vi "demo1.vi"() -> ()   [LabVIEW 2025]
uses:
  Simple_calculator/Control 6.ctl
panel:
  out "result":dbl
  in  "operand2":dbl
  in  "operand1":dbl
  in  "Enum":T1
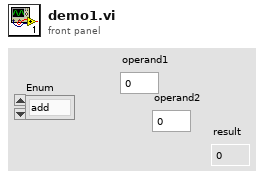
[diagram p1: front panel]
types:
  T1 = typedef "Control 6.ctl" = enum16{"add", "multiply"}
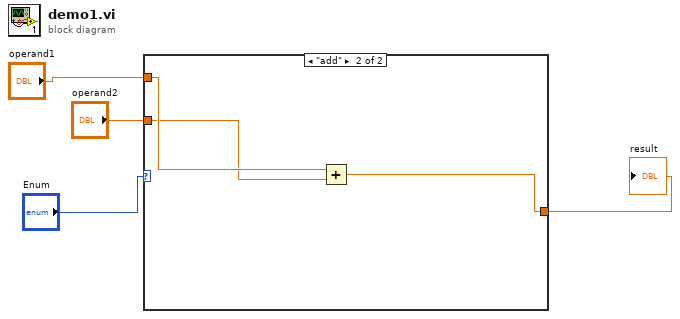
[diagram p0: block diagram]
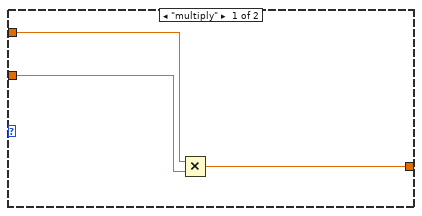
[diagram p2: hidden frame]
diagram:
  n1 = case shown="\"add\"" "Enum" {
    tunnel: "operand1" -> [w7 w10]
    tunnel: "operand2" -> [w6 w9]
    tunnel: [w5 w8] -> w1
    frame "multiply" {
      n2 = Multiply(x=w7, y=w6) -> (x*y=w5:dbl)
    }
    frame "add" {
      n3 = Add(x=w10, y=w9) -> (x+y=w8:dbl)
    }
  }
  "result" <- w1
